vi "Tick Minor Count Write.vi"(4 "error in (no error)":errorcluster, 5 "Value":u16, 6 "Container State":T3, 7 "Display State In":T1) -> (0 "error out":errorcluster, 3 "Display State Out":T1)   [LabVIEW 2020, in "3D Scatter.xctl"]
uses:
  <vilib>/Math Plots/3D Math Plots/3D Scatter/3D Scatter XCtrl/3D Scatter.xctl
  <vilib>/_xctls/Container State.ctl
  <vilib>/Math Plots/3D Math Plots/3D Scatter/3D Scatter XCtrl/State.ctl
  <vilib>/Math Plots/3D Math Plots/3D Scatter/3D Scatter/3D Scatter.lvclass
  e:/builds/penguin/labview/branches/2020/dev/dist/vi.lib/Math Plots/3D Math Plots/3D Plot/3D Plot/3D Plot.lvclass
  <vilib>/Math Plots/3D Math Plots/3D Plot/Action String/3DMathPlot Ctrl Act Queue.ctl
  <vilib>/Math Plots/3D Math Plots/3D Plot/Action String/3DMathPlot Ctrl Act Cluster.ctl
  <vilib>/Math Plots/3D Math Plots/3D Plot/Action String/3DMathPlot State Class.ctl
  <vilib>/Math Plots/3D Math Plots/3D Plot/3D Plot/3D Plot.lvclass
  <vilib>/_xctls/XControlSupport.lvlib
panel:
  # "Replace the Value Control below with a Control of desired type.\nDo not remove this Control or the others from the connector pane.\nDo not change the connector pane pattern.\nThe Value control should always be the third terminal from top on the input side in the connector pane."
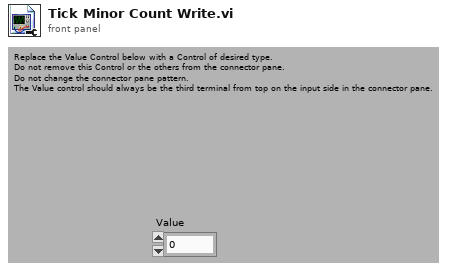
[diagram p1: front panel]
types:
  T1 = typedef "3D Scatter.xctl/State.ctl" = cluster{"3D Scatter.lvclass":refnum<class "3D Scatter.lvclass">, "Control Ref Queue":T2, "Main Frame Color":u32, "Ramp Palette Color":u32, "Projection Palette Color":u32}
  T2 = typedef "3DMathPlot Ctrl Act Queue.ctl" = refnum<queue>
  T3 = typedef "XControlSupport.lvlib/Container State.ctl" = cluster{"Indicator?":bool, "Run Mode?":bool, " Refnum":refnum<vi>}
  T4 = typedef "3DMathPlot State Class.ctl" = enum16{"Update All Objects (Undo)", "Update Light Object Only", "Update Axis Object Only", "Update Plot Object Only", "Update Cursor Object Only", "Update Axis Plot Cursor Objects", "No Update"}
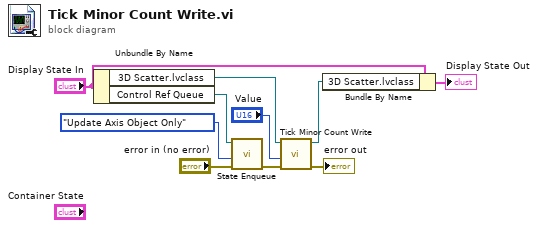
[diagram p0: block diagram]
diagram:
  n1 = Unbundle By Name("Display State In") -> ("3D Scatter.lvclass"=w10:refnum<class "3D Scatter.lvclass">, "Control Ref Queue"=w3:T2)
  n2 = call <vilib>:"State Enqueue.vi"("error in (no error)"="error in (no error)", "Display State Change Class"=3DMathPlot_State_Class."Update Axis Object Only", "Control Ref Queue"=w3) -> ("error out"=w1:errorcluster)  [unwired: 8 out]
  n3 = call <vilib>:"Tick Minor Count Write.vi"("error in (no error)"=w1, "Tick Minor Count"="Value", "3D Plot.lvclass in"=w10) -> ("error out"=→"error out":errorcluster, "3D Plot.lvclass out"=w9:refnum<class "3D Scatter.lvclass">)  [unwired: 7 out]
  n4 = Bundle By Name(cluster="Display State In", "3D Scatter.lvclass"=w9) -> (→"Display State Out":T1)
